vi "Write to Measurement File.vi"   [LabVIEW 2023]
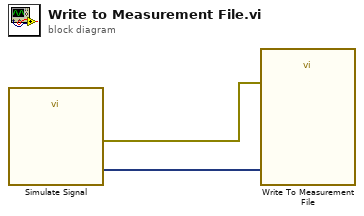
[diagram p0: block diagram]
diagram:
  n1 = call "Simulate Signal"() -> ("Sine"=w2:dynamicdata, "error out"=w1:errorcluster)  [unwired: 14 in]
  n2 = call "Write To Measurement File"("Signals"=w2, "error in (no error)"=w1) -> ()  [unwired: 15 in, 3 out]
